vi "调试专用.vi"   [LabVIEW 2016, in "综合生物毒性.lvlib"]
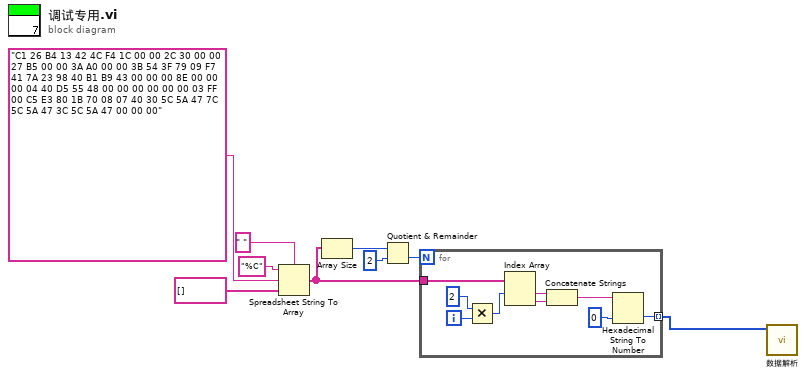
[diagram p0: block diagram]
diagram:
  n1 = Spreadsheet String To Array(delimiter (Tab)=" " ("分隔符(Tab)"), format string="%C" ("格式字符串"), spreadsheet string="C1 26 B4 13 42 4C F4 1C 00 00 2C 30 00 00 27 B5 00 00 3A A0 00 00 3B 54 3F 79 09 F7 41 7A 23 98 40 B1 B9 43 00 00 00 8E 00 00 00 04 40 D5 55 48 00 00 00 00 00 00 03 FF 00 C5 E3 80 1B 70 08 07 40 30 5C 5A 47 7C 5C 5A 47 3C 5C 5A 47 00 00 00", array type (2D Dbl)=string[] []) -> (array=w3:string[])
  n2 = Array Size(array=w3) -> (size(s)=w5:i32)
  n3 = Quotient & Remainder(x=w5, y=2) -> (floor(x/y)=w2:i32)  [unwired: 1 out]
  n4 = for {
    N: w2 -> [_]
    tunnel: w3 -> [w15]
    tunnel: [w10] -> w1 mode=indexing
    i -> [w18]
    n5 = Multiply(x=2, y=w18) -> (x*y=w16:i32)
    n6 = Index Array(array=w15, index #1=w16) -> (element #1=w13:string, element #2=w14:string)  [unwired: 1 in]
    n7 = Concatenate Strings(w13, w14) -> (w12:string)
    n8 = Hexadecimal String To Number(string=w12, default (0uL)=u16 0 ("默认(0 U32)")) -> (number=w10:u16)  [unwired: 1 in, 1 out]
  }
  n9 = call "数据解析.vi"("数组"=w1) -> ()  [unwired: 10 in, 1 out]
